vi "ws_editscenario Export Scenario.vi"(8 "error in (no error)":errorcluster, 10 "sxScenarioId (\"\")":string, 11 "Connection Refnum":T1) -> (0 "error out":errorcluster, 2 "scenario XML":string, 3 "Connection Refnum":T1)   [LabVIEW 2011]
uses:
  SI.LIB/ODBC/SQL Controls/Connection Refnum.ctl
  scenario xml.ctl
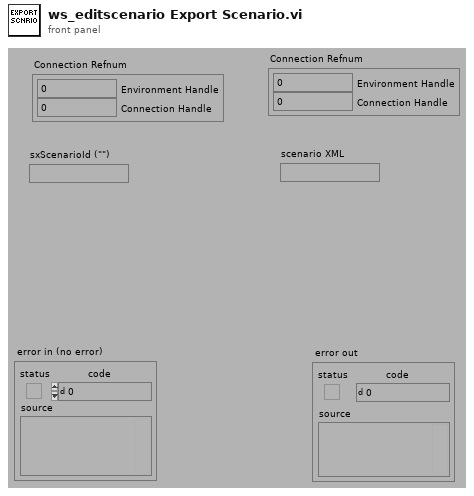
[diagram p1: front panel]
types:
  T1 = typedef "Connection Refnum.ctl" = cluster{"Environment Handle":i32, "Connection Handle":i32}
  T2 = typedef "scenario xml.ctl" = cluster{"#attributes":cluster{"version":string, "creator":string}, "sxScenarioId":string, "sDescription":string, "sLogic":string, "sResultFieldsCSV":string, "sTemplatesCSV":string, "fAutoRunReports":bool, "fSortByTemplates":bool, "fCombinePDF":bool, "Conditions":cluster{"sxFieldId":string, "nOperator":string, "sMatchValue":string}[]}
  T3 = typedef "OGAB Version.ctl" = cluster{"Version":string, "Build Number":u32, "Build Date/Time":dbl}
  T4 = typedef "Scenario Record.ctl" = cluster{"ixScenario":i32, "tCreated":timestamp, "tModified":timestamp, "sxUsername":string, "sModifiedBy":string, "sxScenarioId":string, "sDescription":string, "sLogic":string, "sResultFieldsCSV":string, "sTemplatesCSV":string, "fAutoRunReports":bool, "fSortByTemplates":bool, "fCombinePDF":bool, "Conditions":T5[]}
  T5 = typedef "Condition Record.ctl" = cluster{"iConditionIndex":i32, "sxFieldId":string, "nOperator":T6, "sMatchValue":string}
  T6 = typedef "Condition Operators.ctl" = enum16{"equal (=)", "not equal (\\u2260)", "less than (<)", "less than or equal (\\u2264)", "greater than (>)", "greater than or equal (\\u2265)", "contains", "does not contain"}
  T7 = cluster{"sxFieldId":string, "nOperator":string, "sMatchValue":string}[]
  T8 = cluster{"sxFieldId":string, "nOperator":string, "sMatchValue":string}
  T9 = typedef "Field Record.ctl" = cluster{"ixField":i32, "iSequenceOrder":i32, "sxFieldId":string, "sxSequenceId":string, "sDisplayName":string, "sValue":string, "sUnits":string, "nDataType":T10, "nNextItem":T11, "fSystem":bool, "fSystemValue":bool, "fRequired":bool, "fSetAtTest":bool, "fTestField":bool, "fDeleted":bool, "fIndexed":bool, "fFreeList":bool}
  T10 = typedef "Field DataTypes.ctl" = enum32{"text", "numeric", "list", "timestamp", "boolean"}
  T11 = typedef "Field NextItem.ctl" = enum32{"Reset", "Retain", "Auto-Increment"}
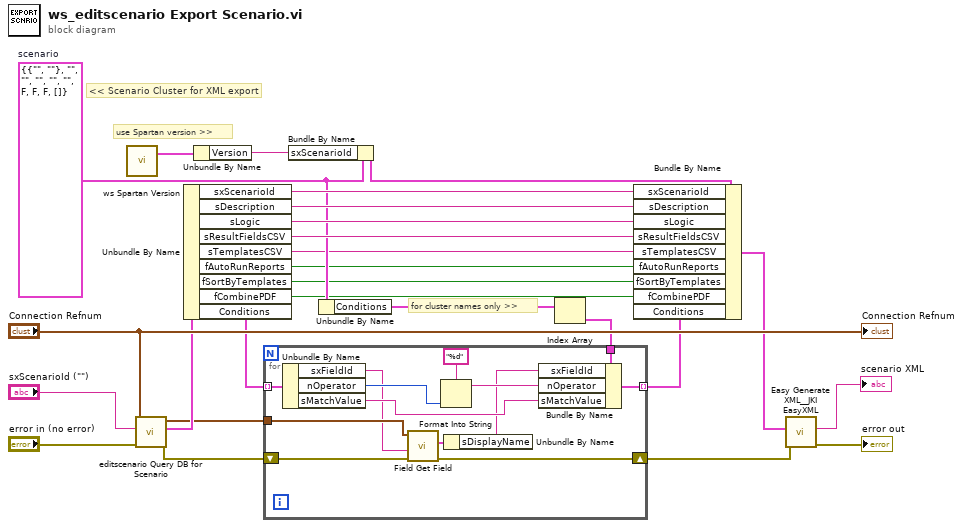
[diagram p0: block diagram]
diagram:
  w13 = T2 {"#attributes"={"version"="", "creator"=""}, "sxScenarioId"="", "sDescription"="", "sLogic"="", "sResultFieldsCSV"="", "sTemplatesCSV"="", "fAutoRunReports"=FALSE, "fSortByTemplates"=FALSE, "fCombinePDF"=FALSE, "Conditions"=[]}  # scenario
  # "use Spartan version >>"
  # "for cluster names only >>"
  # "<< Scenario Cluster for XML export"
  n1 = call "ws Spartan Version.vi"() -> ("Version"=w22:T3)  [unwired: 3 in]
  n2 = call "editscenario Query DB for Scenario.vi"("error in (no error)"="error in (no error)", "sxScenarioId (\"\")"="sxScenarioId (\"\")", "Connection Refnum"="Connection Refnum") -> ("error out"=w6:errorcluster, "Scenario Record"=w23:T4, "Connection Refnum"=w5:T1)  [unwired: 6 out]
  n3 = Unbundle By Name(w23) -> ("sxScenarioId"=w21:string, "sDescription"=w20:string, "sLogic"=w19:string, "sResultFieldsCSV"=w18:string, "sTemplatesCSV"=w7:string, "fAutoRunReports"=w1:bool, "fSortByTemplates"=w3:bool, "fCombinePDF"=w2:bool, "Conditions"=w17:T5[])
  n4 = Unbundle By Name(w22) -> ("Version"=w11:string)
  n5 = Bundle By Name(cluster=w13, "sxScenarioId"=w11) -> (w12:T2)
  n6 = Unbundle By Name(w13) -> ("Conditions"=w9:T7)
  n7 = Index Array(array=w9) -> (element=w8:T8)  [unwired: 1 in]
  n8 = for {
    tunnel: w17 -> [w39] mode=indexing
    tunnel: w8 -> [w38]
    tunnel: [w37] -> w16 mode=indexing
    shift-right: [w27] -> w4
    shift-left: w6 -> [w31]
    tunnel: w5 -> [w32]
    n9 = Unbundle By Name(w39) -> ("sxFieldId"=w30:string, "nOperator"=w35:T6, "sMatchValue"=w36:string)
    n10 = call "Field Get Field.vi"("error in (no error)"=w31, "sFieldId or sDisplayName (\"\")"=w30, "Connection Refnum"=w32) -> ("error out"=w27:errorcluster, "Field"=w29:T9)  [unwired: 2 in, 5 out]
    n11 = Format Into String(format string="%d", w35) -> (resulting string=w33:string)  [unwired: 2 in, 1 out]
    n12 = Unbundle By Name(w29) -> ("sDisplayName"=w28:string)
    n13 = Bundle By Name(cluster=w38, "sxFieldId"=w28, "nOperator"=w33, "sMatchValue"=w36) -> (w37:T8)
  }
  n14 = Bundle By Name(cluster=w12, "sxScenarioId"=w21, "sDescription"=w20, "sLogic"=w19, "sResultFieldsCSV"=w18, "sTemplatesCSV"=w7, "fAutoRunReports"=w1, "fSortByTemplates"=w3, "fCombinePDF"=w2, "Conditions"=w16) -> (w15:T2)
  n15 = call <vilib>:"Easy Generate XML__JKI EasyXML.vi"("error in (no error)"=w4, "LabVIEW Data"=w15) -> ("error out"=→"error out":errorcluster, "XML String"=→"scenario XML":string)  [unwired: 8 out]
  "Connection Refnum" <- "Connection Refnum"
